vi "Read Boolean.vi"(11 "Double Array Event in":refnum<class "Boolean Event.lvclass">) -> (2 "Boolean":bool, 3 "Double Array Event out":refnum<class "Boolean Event.lvclass">)   [LabVIEW 2016, in "Boolean Event.lvclass"]
uses:
  Boolean Event.lvclass
  Boolean Event.lvclass/Boolean Event.ctl
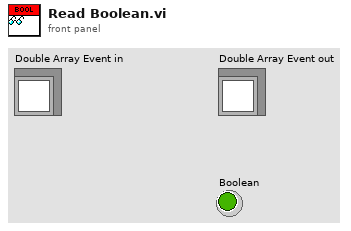
[diagram p1: front panel]
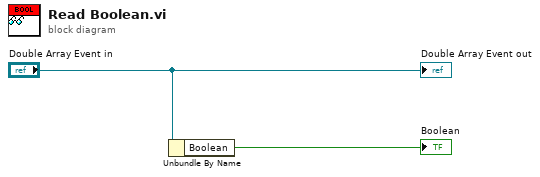
[diagram p0: block diagram]
diagram:
  n1 = Unbundle By Name("Double Array Event in") -> ("Boolean"=→"Boolean":bool)
  "Double Array Event out" <- "Double Array Event in"
